vi "PCert-Container-ConstructMemCont.vi"(8 "error in (no error)":errorcluster, 11 "ERP-Container-UI in":refnum<class "PCert-Container-UI.lvclass">) -> (0 "error out":errorcluster, 3 "ERP-Container-UI out":refnum<class "PCert-Container-UI.lvclass">)   [LabVIEW 2013, in "PCert-Container-UI.lvclass"]
uses:
  PCert-Container-UI.lvclass
  PCert-Container-UI.lvclass/PCert-Container-UI.ctl
  ftw-dataflow/Core/src/Database/FTW-SQLite-DatabaseType.ctl
  ftw-dataflow/Core/src/Database/FTW-SQLite-Connector.lvclass
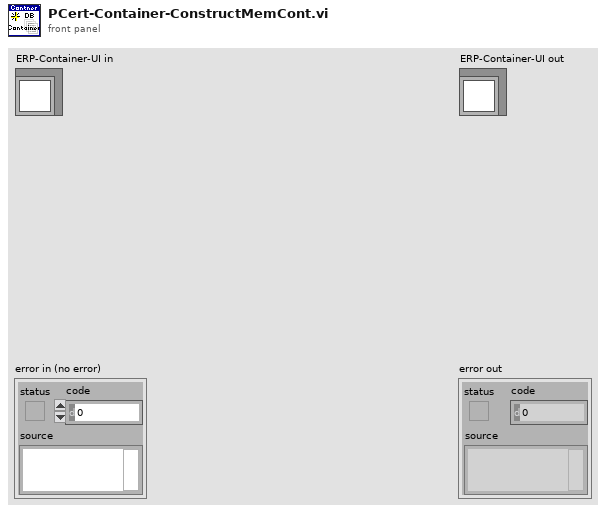
[diagram p1: front panel]
types:
  T1 = typedef "FTW-SQLite-Connector.lvclass/FTW-SQLite-DatabaseType.ctl" = enum16{"Disk", "Memory"}
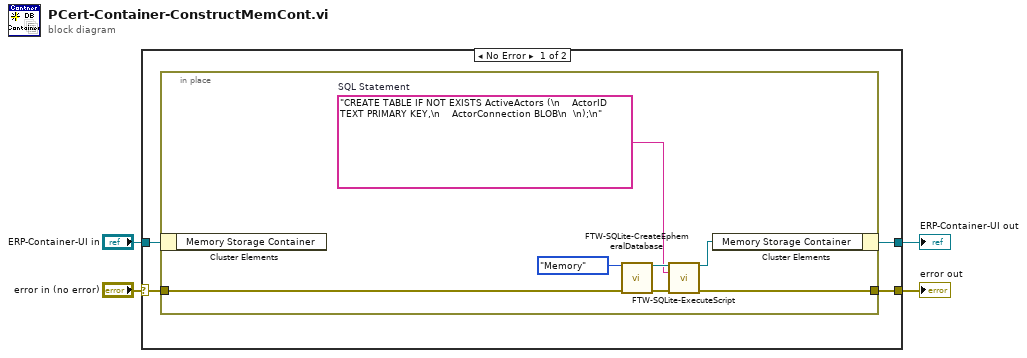
[diagram p0: block diagram]
diagram:
  n1 = case shown="No Error" "error in (no error)" {
    selector: "error in (no error)" -> [w6 w17]
    tunnel: [w5 w17] -> w3
    tunnel: [w7 w16] -> w1
    tunnel: "ERP-Container-UI in" -> [w8 w16]
    frame No Error {
      n2 = in-place {
        in-place-border: w6 -> [w10]
        in-place-border: [w9] -> w5
        w13 = "CREATE TABLE IF NOT EXISTS ActiveActors (\n    ActorID TEXT PRIMARY KEY,\n    ActorConnection BLOB\n  \n);\n"  # SQL Statement
        n3 = in-place-cluster #1(w8) -> ()  [unwired: 1 out]
        n4 = call "FTW-SQLite-CreateEphemeralDatabase.vi"("Database Type"=FTW-SQLite-DatabaseType."Memory", "error in"=w10) -> ("SQLite Connector"=w14:refnum<class "FTW-SQLite-Connector.lvclass">, "error out"=w12:errorcluster)  [unwired: 12 in]
        n5 = call "FTW-SQLite-ExecuteScript.vi"("SQLite Connector"=w14, "SQL Script"=w13, "error in"=w12) -> ("SQLite Connector out"=w11:refnum<class "FTW-SQLite-Connector.lvclass">, "error out"=w9:errorcluster)  [unwired: 9 in, 2 out]
        n6 = in-place-cluster #1("Memory Storage Container"=w11) -> (w7:refnum<class "PCert-Container-UI.lvclass">)
      }
    }
    frame Error {
    }
  }
  "error out" <- w3
  "ERP-Container-UI out" <- w1
